vi "get_rep_param.vi"(4 "error in (no error)":errorcluster, 6 "param_name":string, 7 "refnum":T1) -> (0 "error out":errorcluster, 1 "list":string[](array[string]), 2 "default":i32, 3 "refnum out":T1)   [LabVIEW 2010]
uses:
  <vilib>/Utility/config.llb/Config Data RefNum.ctl
  <vilib>/Utility/config.llb/Write Key (I32).vi
  <vilib>/Utility/config.llb/Write Key (String).vi
  <vilib>/Utility/config.llb/Read Key (I32).vi
  <vilib>/Utility/config.llb/Read Key (String).vi
  <vilib>/Utility/config.llb/NI_LVConfig.lvlib
panel:
  in  "par_val":string
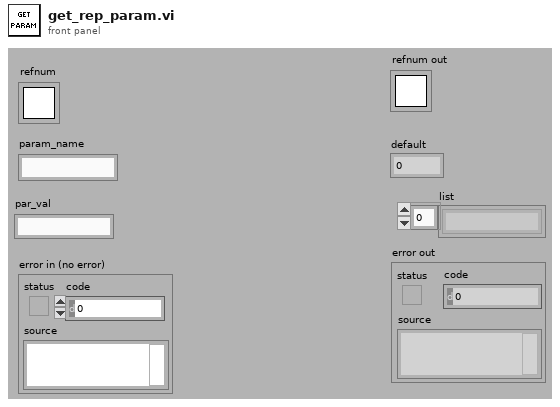
[diagram p1: front panel]
types:
  T1 = typedef "NI_LVConfig.lvlib/Config Data RefNum.ctl" = refnum<k1>
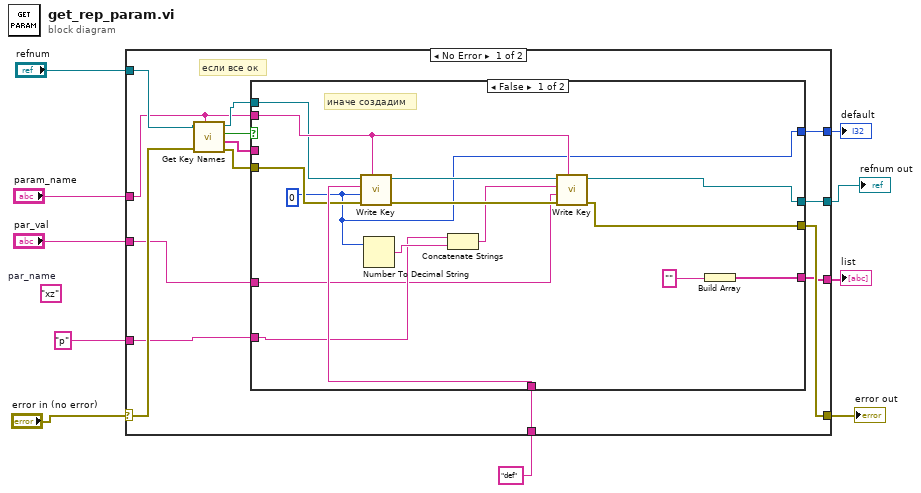
[diagram p0: block diagram]
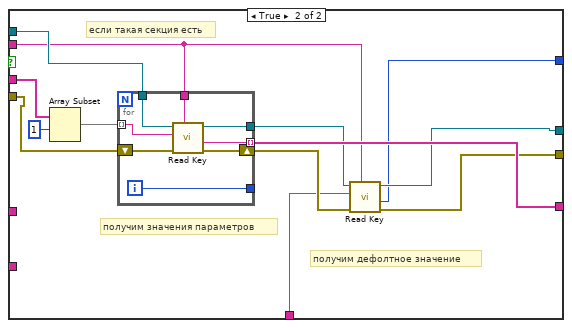
[diagram p2: hidden frame]
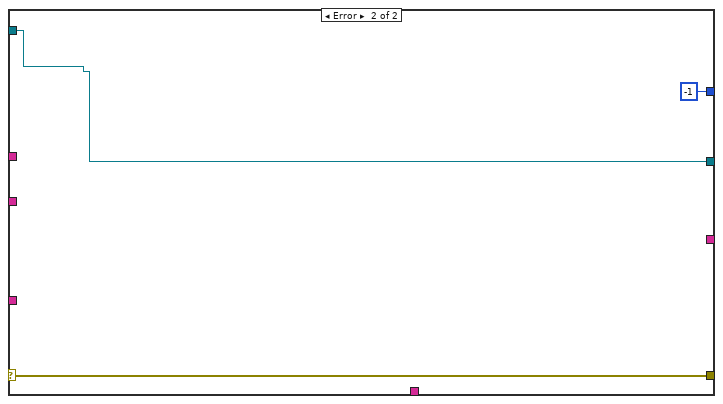
[diagram p3: hidden frame]
diagram:
  (unwired) "xz"  # par_name
  n1 = case shown="No Error" "error in (no error)" {
    selector: "error in (no error)" -> [w24 w63]
    tunnel: [w14 w63] -> w9
    tunnel: "refnum" -> [w23 w62]
    tunnel: "param_name" -> [w17 _]
    tunnel: "p" -> [w18 _]
    tunnel: "par_val" -> [w16 _]
    tunnel: "def" -> [w15 _]
    tunnel: [w13 w62] -> w3
    tunnel: [w12 _] -> w2
    tunnel: [w11 -1 ("value")] -> w1
    frame No Error {
      # "если все ок"
      n2 = call <vilib>:"Get Key Names.vi"("section"=w17, "error in (no error)"=w24, "refnum"=w23) -> ("error out"=w21:errorcluster, "key names"=w19:string[], "section exists?"=w22:bool, "refnum out"=w20:T1)  [unwired: 5 in]
      n3 = case shown="False" w22 {
        tunnel: w21 -> [w29 w50]
        tunnel: w20 -> [w36 w48]
        tunnel: w19 -> [_ w52]
        tunnel: w18 -> [w31 _]
        tunnel: w17 -> [w37 w42]
        tunnel: w16 -> [w26 _]
        tunnel: w15 -> [w33 w41]
        tunnel: [w34 w45] -> w14
        tunnel: [w35 w44] -> w13
        tunnel: [w27 w47] -> w12
        tunnel: [w28 w40] -> w11
        frame False {
          w28 = 0
          # "иначе создадим"
          n4 = call-poly <vilib>:"Write Key.vi"("section"=w37, "error in (no error)"=w29, "value"=w28, "key"=w33, "refnum"=w36) -> ("error out"=w39:errorcluster, "refnum out"=w38:T1)  [unwired: 4 in, 1 out]
          n5 = Number To Decimal String(number=w28) -> (decimal integer string=w32:string)  [unwired: 1 in]
          n6 = Concatenate Strings(w31, w32) -> (w30:string)
          n7 = call-poly <vilib>:"Write Key.vi"("section"=w37, "error in (no error)"=w39, "value"=w26, "key"=w30, "refnum"=w38) -> ("error out"=w34:errorcluster, "refnum out"=w35:T1)  [unwired: 4 in, 1 out]
          n8 = Build Array("") -> (w27:string[])
        }
        frame True {
          # "получим дефолтное значение"
          # "получим значения параметров"
          # "если такая секция есть"
          n9 = Array Subset(array=w52, index=1) -> (w49:string[])  [unwired: 1 in]
          n10 = for {
            tunnel: w49 -> [w57] mode=indexing
            tunnel: w42 -> [w59]
            tunnel: w48 -> [w58]
            tunnel: [w55] -> w43
            tunnel: [w54] -> w47 mode=indexing
            shift-right: [w56] -> w46
            shift-left: w50 -> [w60]
            tunnel: [w53] -> _
            i -> [w53]
            n11 = call-poly <vilib>:"Read Key.vi"("section"=w59, "error in (no error)"=w60, "key"=w57, "refnum"=w58) -> ("error out"=w56:errorcluster, "value"=w54:string, "refnum out"=w55:T1)  [unwired: 4 in, 1 out]
          }
          n12 = call-poly <vilib>:"Read Key.vi"("section"=w42, "error in (no error)"=w46, "key"=w41, "refnum"=w43) -> ("error out"=w45:errorcluster, "value"=w40:i32, "refnum out"=w44:T1)  [unwired: 4 in, 1 out]
        }
      }
    }
    frame Error {
    }
  }
  "error out" <- w9
  "refnum out" <- w3
  "list" <- w2
  "default" <- w1
